vi "Read_Temperature.vi"(11 "Temperature sensor Channel":tag) -> (0 "Temperature":dbl, 1 "voltage 4":dbl(knob) scale=0.0..100.0, 2 "voltage 3":dbl(knob) scale=0.0..5.0, 3 "voltage 2":dbl(knob) scale=0.0..5.0)   [LabVIEW 2022 SP3]
uses:
  <vilib>/DAQmx/read.llb/DAQmx Read (Analog Wfm 1Chan 1Samp).vi
  <vilib>/DAQmx/create/channels.llb/DAQmx Create Channel (AI-Voltage-Basic).vi
  <vilib>/DAQmx/miscellaneous.llb/DAQmx Fill In Error Info.vi
  <vilib>/ptbypt/NI_PtbyPt.lvlib
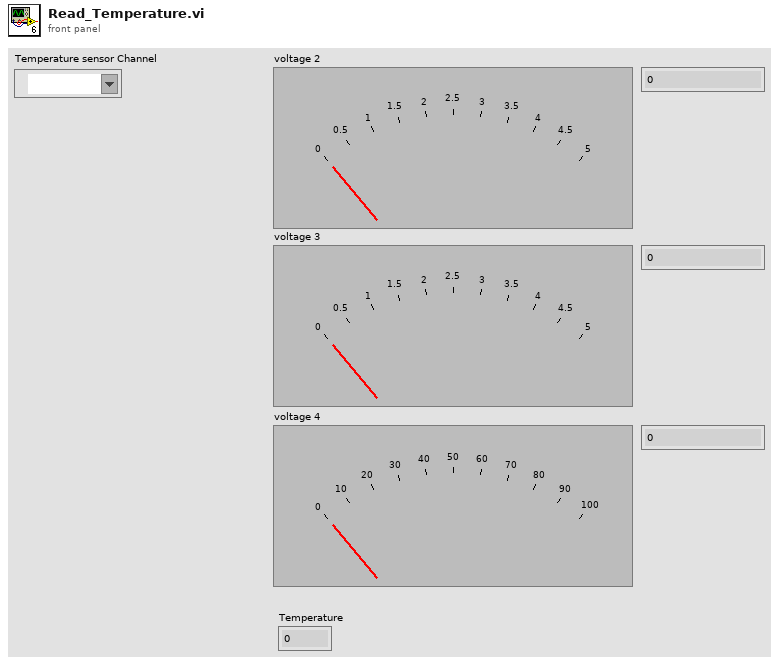
[diagram p1: front panel]
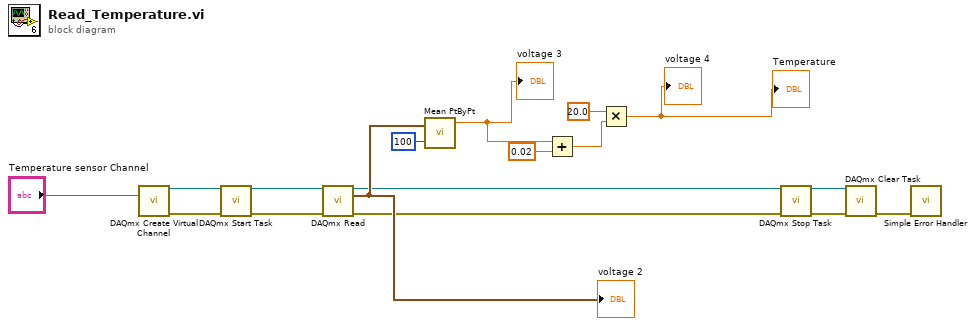
[diagram p0: block diagram]
diagram:
  n1 = call-poly <vilib>:"DAQmx Create Virtual Channel.vi"("physical channels"="Temperature sensor Channel") -> ("task out"=w13:refnum<k21>, "error out"=w12:errorcluster)  [unwired: 13 in]
  n2 = call <vilib>:"DAQmx Start Task.vi"("task/channels in"=w13, "error in"=w12) -> ("task out"=w5:refnum<k21>, "error out"=w4:errorcluster)  [unwired: 12 in]
  n3 = call-poly <vilib>:"DAQmx Read.vi"("task/channels in"=w5, "error in"=w4) -> ("task out"=w3:refnum<k21>, "data"=w11:waveform(dbl), "error out"=w2:errorcluster)  [unwired: 11 in]
  "voltage 2" <- w11
  n4 = call <vilib>:"Mean PtByPt.vi"("x"=w11, "sample length"=100) -> ("mean"=w8:dbl)  [unwired: 2 in, 1 out]
  "voltage 3" <- w8
  n5 = Add(x=w8, y=0.02) -> (x+y=w7:dbl)
  n6 = Multiply(x=20.0, y=w7) -> (x*y=→"voltage 4" →"Temperature":dbl)
  n7 = call <vilib>:"DAQmx Stop Task.vi"("task/channels in"=w3, "error in"=w2) -> ("task out"=w16:refnum<k21>, "error out"=w15:errorcluster)  [unwired: 12 in]
  n8 = call <vilib>:"DAQmx Clear Task.vi"("task in"=w16, "error in"=w15) -> ("error out"=w17:errorcluster)  [unwired: 13 in]
  n9 = call <vilib>:"Simple Error Handler.vi"("error in (no error)"=w17) -> ()  [unwired: 4 in, 5 out]
